vi "Leaderboard test 3.vi"() -> ()   [LabVIEW 2020, in "Visualisation.lvclass"]
uses:
  Visualisation.lvclass
  Application/Globals.vi
  Data Manager/Data Manager.lvclass
  Application/Application.lvlib
panel:
  out "Leaderboard":T1(array[cluster]) {"Distance 3"."Distance 4" scale=0.0..12.161000000000001; "Distance 3"."Distance 3" scale=0.0..42.4483; "Distance 3"."Distance 2" scale=0.0..37.579899999999995; "Distance" format="%#.1f km"}
  out "B Total":dbl format="%0.1f km"
  out "A Total":dbl format="%0.1f km"
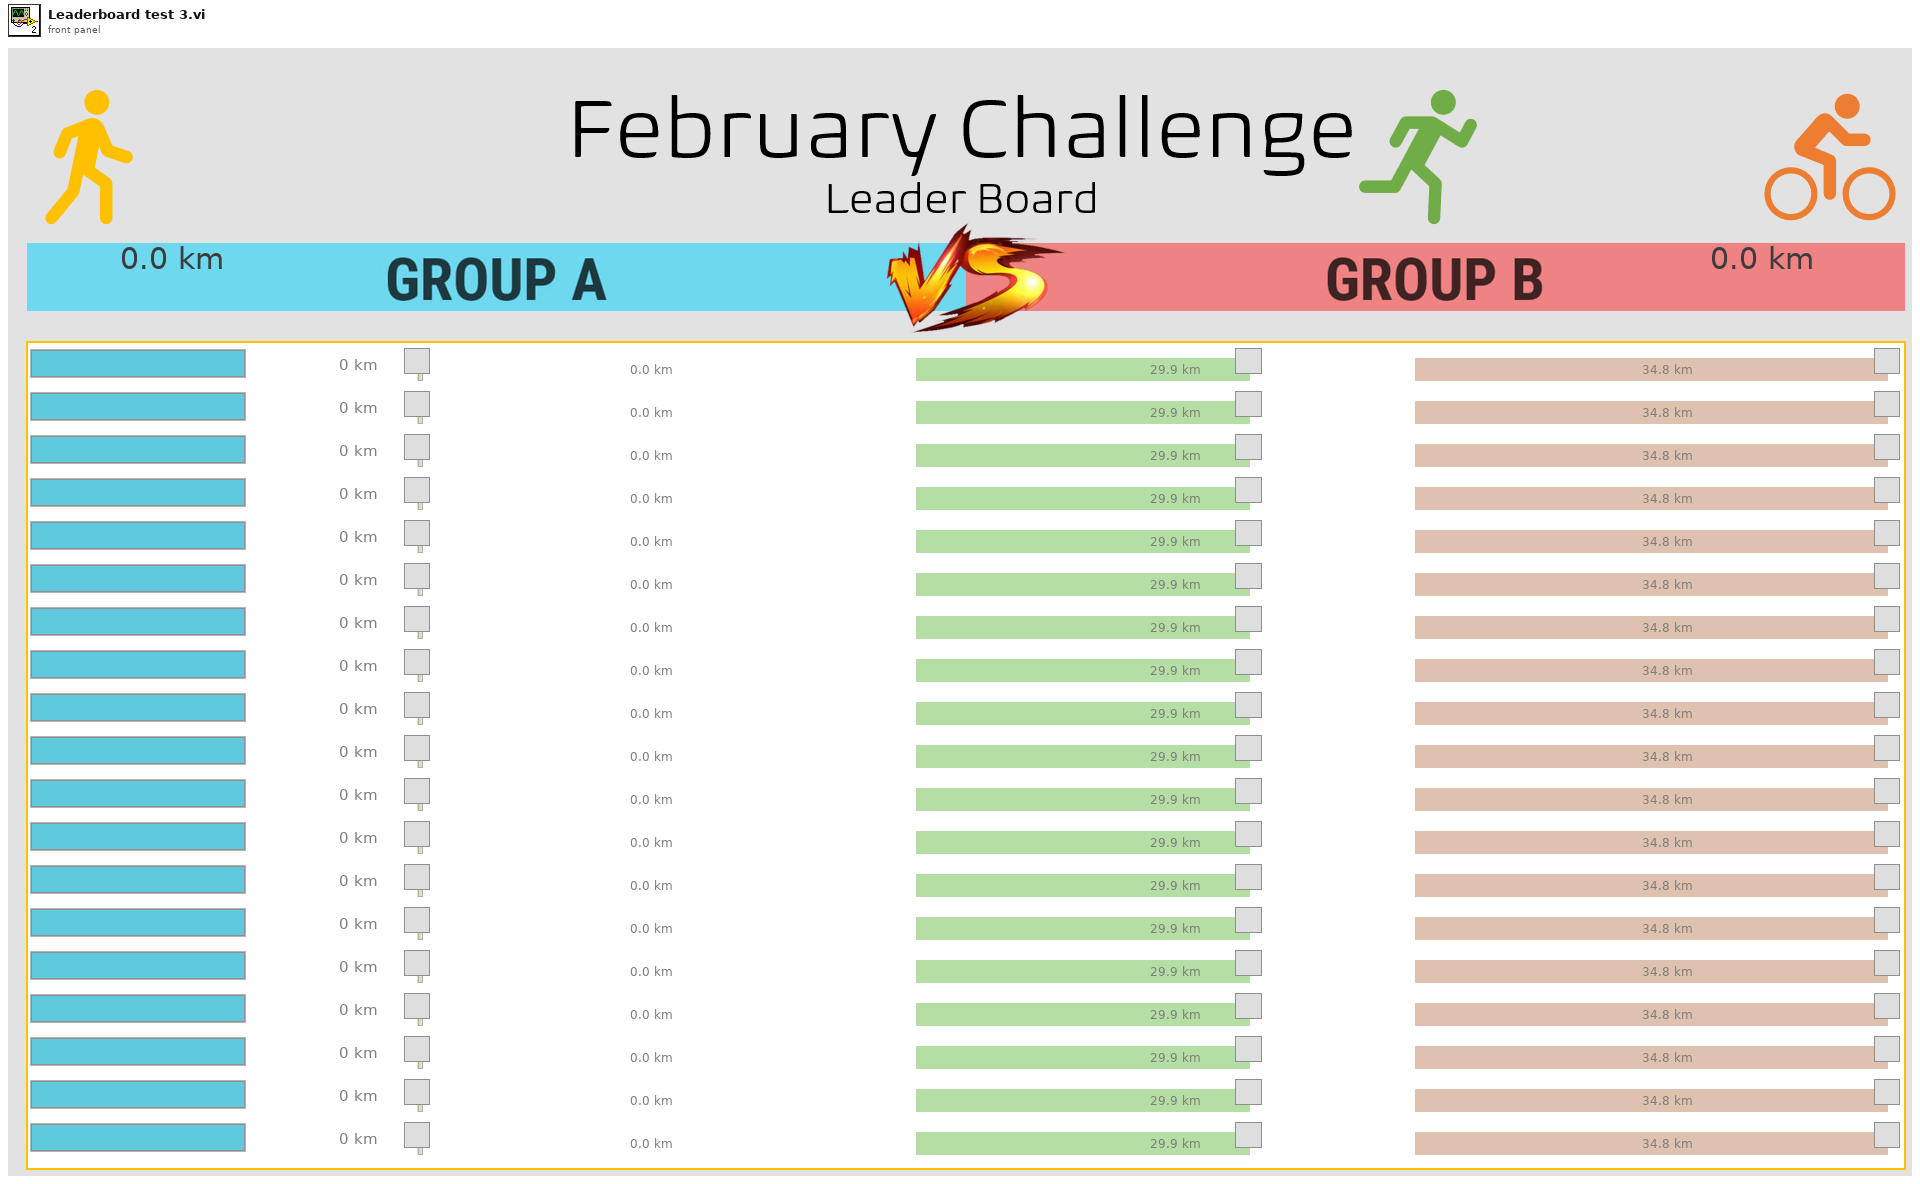
[diagram p1: front panel]
types:
  T1 = cluster{"Athlete":string, "Distance":dbl, "Team":u32, "Distance 3":cluster{"Distance 2":dbl, "Distance 3":dbl, "Distance 4":dbl}}[]
  T2 = cluster{"Athlete":string, "Distance":dbl, "Team":u32, "Distance 2":cluster{"Numeric":dbl, "Numeric":dbl, "Numeric":dbl}}
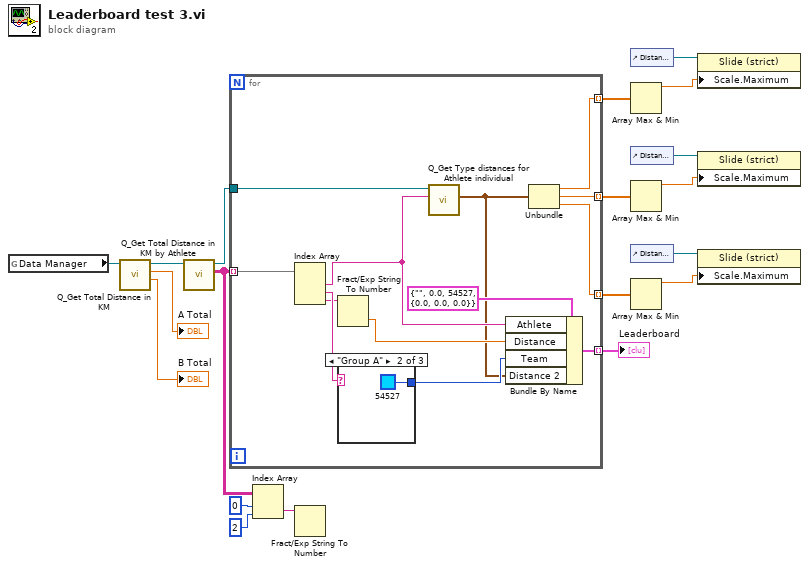
[diagram p0: block diagram]
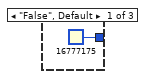
[diagram p2: hidden frame]
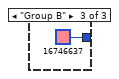
[diagram p3: hidden frame]
diagram:
  n1 = global read "Globals.vi" "Data Manager"() -> (w19:refnum<class "Data Manager.lvclass">)
  n2 = call-dynamic "Q_Get Total Distance in KM.vi"("Data Manager in"=w19) -> ("Group B"=→"B Total":dbl, "Group A"=→"A Total":dbl, "Data Manager out"=w16:refnum<class "Data Manager.lvclass">)  [unwired: 6 in, 2 out]
  n3 = call-dynamic "Q_Get Total Distance in KM by Athlete.vi"("Data Manager in"=w16) -> ("Result Set"=w11:string[][], "Data Manager out"=w10:refnum<class "Data Manager.lvclass">)  [unwired: 8 in, 1 out]
  n4 = for {
    tunnel: w11 -> [w30] mode=indexing
    tunnel: [w31] -> w13 mode=indexing
    tunnel: w10 -> [w22]
    tunnel: [w25] -> w4 mode=indexing
    tunnel: [w24] -> w5 mode=indexing
    tunnel: [w23] -> w6 mode=indexing
    n5 = Index Array(array=w30) -> (element #1=w21:string, element #2=w27:string, element #3=w26:string)  [unwired: 3 in]
    n6 = Fract/Exp String To Number(string=w26) -> (number=w29:dbl)  [unwired: 3 in, 1 out]
    n7 = case shown="\"Group A\"" w27 {
      tunnel: [u32 16777175 ("Color Box") u32 54527 ("Color Box") u32 16746637 ("Color Box")] -> w28
      frame "False", Default {
      }
      frame "Group A" {
      }
      frame "Group B" {
      }
    }
    n8 = call-dynamic "Q_Get Type distances for Athlete individual.vi"("Alias"=w21, "Data Manager in"=w22) -> ("output cluster"=w20:cluster{dbl, dbl, dbl})  [unwired: 6 in, 3 out]
    n9 = Bundle By Name(cluster=T2 {"Athlete"="", "Distance"=0.0, "Team"=54527, "Distance 2"={"Numeric"=0.0, "Numeric"=0.0, "Numeric"=0.0}} ("Leaderboard"), "Athlete"=w21, "Distance"=w29, "Team"=w28, "Distance 2"=w20) -> (w31:T2)
    n10 = Unbundle(w20) -> (w25:dbl, w24:dbl, w23:dbl)
  }
  "Leaderboard" <- w13
  n11 = Index Array(array=w11, index (row)=0, index (col)=2 ("disabled index (col)")) -> (element=w12:string)
  n12 = Fract/Exp String To Number(string=w12) -> ()  [unwired: 3 in, 2 out]
  n13 = control-ref of="Distance 2"() -> (w9:refnum<vi>)
  n14 = Array Max & Min(array=w4) -> (max value=w3:dbl)  [unwired: 3 out]
  n15 = control-ref of="Distance 3"() -> (w8:refnum<vi>)
  n16 = Array Max & Min(array=w5) -> (max value=w2:dbl)  [unwired: 3 out]
  n17 = control-ref of="Distance 4"() -> (w7:refnum<vi>)
  n18 = Array Max & Min(array=w6) -> (max value=w1:dbl)  [unwired: 3 out]
  n19 = property on="Property Node" class="Slide (strict)"(reference=w9, "Scale.Maximum"=w3) -> ()  [unwired: 1 in, 2 out]
  n20 = property on="Property Node" class="Slide (strict)"(reference=w8, "Scale.Maximum"=w2) -> ()  [unwired: 1 in, 2 out]
  n21 = property on="Property Node" class="Slide (strict)"(reference=w7, "Scale.Maximum"=w1) -> ()  [unwired: 1 in, 2 out]
